vi "Lab 9 Exercise 4 - Using Loops.vi"() -> ()   [LabVIEW 2023]
panel:
  out "Waveform Chart":dbl(graph)
  in  "stop":bool
  in  "Millisecond Delay":dbl(slide) scale=0.0..10.0
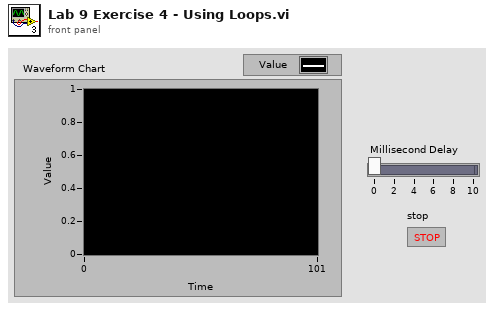
[diagram p1: front panel]
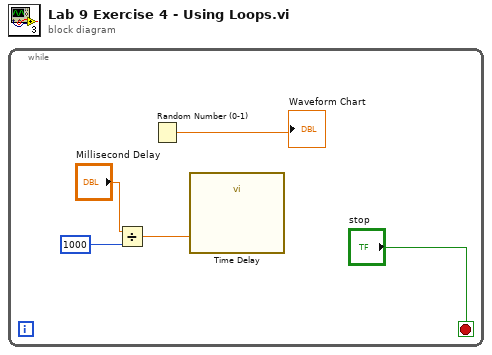
[diagram p0: block diagram]
diagram:
  n1 = while {
    stop <- "stop" stop-if-true
    n2 = Divide(x="Millisecond Delay", y=1000) -> (x/y=w1:dbl)
    n3 = Random Number (0-1)() -> (number: 0 to 1=→"Waveform Chart":dbl)
    n4 = call "Time Delay"("Delay Time (s)"=w1) -> ()  [unwired: 10 in, 1 out]
  }
